vi "Send Command String.vi"(8 "error in (no error)":errorcluster, 10 "Send Command String":string, 11 "VISA resource name":refnum<visa-resource-name>) -> (0 "error out":errorcluster, 3 "VISA resource name out":refnum<visa-resource-name>)   [LabVIEW 2023, in "Fluke Molbox 1 Plus.lvlib"]
doc: "Sends a command string to communicate with a device connected to the molbox1+ COM2 port. The molbox1+ COM2 port can be used to communicate to another RS232 device (e.g., another molbox1+ or a multimeter). This allows the user to use one COM port or IEEE-488 port on the host computer to communicate with the molbox1+ and another device. A carriage return and a line feed (<CR><LF>) are added to the string."
uses:
  Fluke Molbox 1 Plus.lvlib
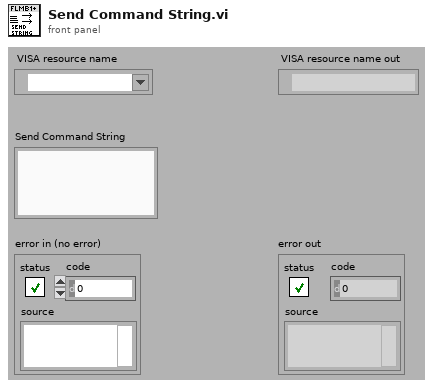
[diagram p1: front panel]
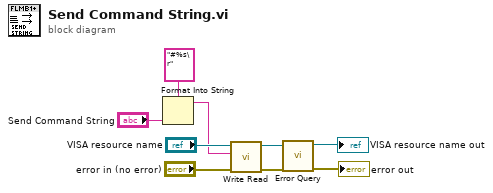
[diagram p0: block diagram]
diagram:
  n1 = Format Into String(format string="#%s\r", "Send Command String") -> (resulting string=w6:string)  [unwired: 2 in, 1 out]
  n2 = call "Write Read.vi"("error in (no error)"="error in (no error)", "Write String"=w6, "VISA resource name"="VISA resource name") -> ("error out"=w3:errorcluster, "VISA resource name out"=w4:refnum<visa-resource-name>)  [unwired: 6 in, 1 out]
  n3 = call "Error Query.vi"("error in (no error)"=w3, "VISA resource name"=w4) -> ("error out"=→"error out":errorcluster, "VISA resource name out"=→"VISA resource name out":refnum<visa-resource-name>)  [unwired: 6 in, 2 out]
